vi "Build FIU Section from XML.vi"(6 "Channels":refnum<k24>[](array[refnum]), 8 "error in (no error)":errorcluster, 9 "Card Position in":T1 {"Slot #" max=15}, 10 "Name in":string, 11 "Node Ptr in":u64) -> (0 "error out":errorcluster)   [LabVIEW 2014, in "SLSC configuration System Explorer.lvlib"]
uses:
  SLSC configuration System Explorer.lvlib
  Type Defs/Card Position.ctl
  Shared/SPI Utility/Slot #.ctl
  <vilib>/NI Veristand/Custom Device API/Custom Device Channel.ctl
  <vilib>/NI Veristand/Custom Device API/Custom Device Channel Type.ctl
  Shared/Constants.vi
  <vilib>/NI Veristand/Custom Device API/Set Item Property (U16).vi
  <vilib>/NI Veristand/Custom Device API/Custom Device API.lvlib
  Shared/SLSC configuration Shared.lvlib
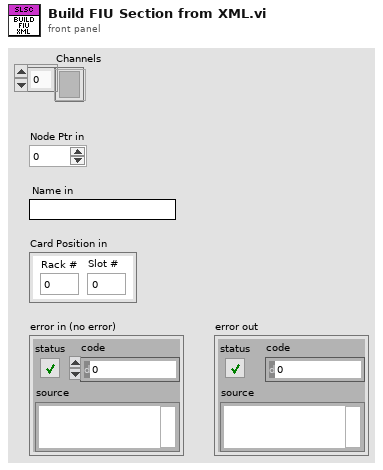
[diagram p1: front panel]
types:
  T1 = typedef "SLSC configuration Shared.lvlib/Card Position.ctl" = cluster{"Rack #":u8, "Slot #":T2}
  T2 = typedef "SLSC configuration Shared.lvlib/Slot #.ctl" = u8
  T3 = typedef "Custom Device API.lvlib/Custom Device Channel Type.ctl" = enum16{"Input", "Output"}
  T4 = typedef "Custom Device API.lvlib/Custom Device Channel.ctl" = cluster{"Type":T3, "Units":string, "Default Value":dbl, "Faultable":bool, "Scalable":bool}
  T5 = typedef "Custom Device API.lvlib/Custom Device Item Ref.ctl" = u64
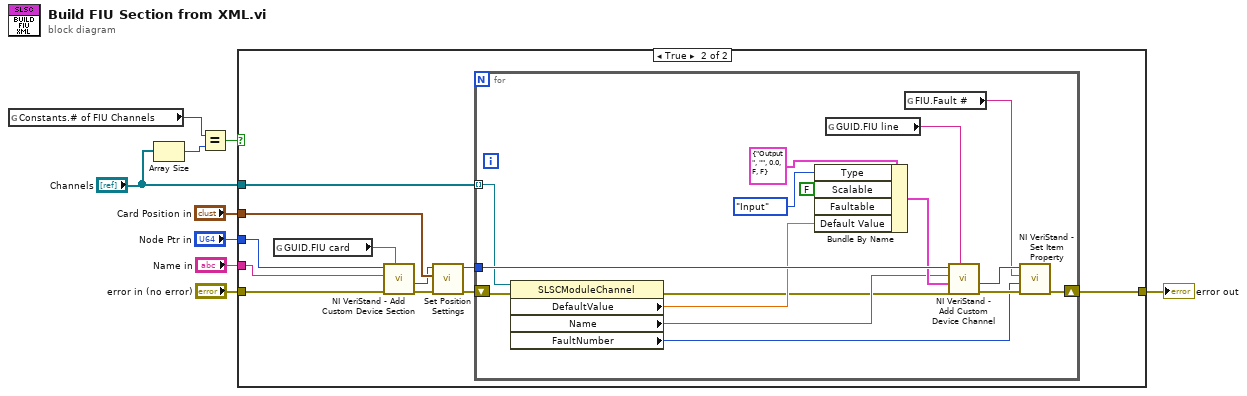
[diagram p0: block diagram]
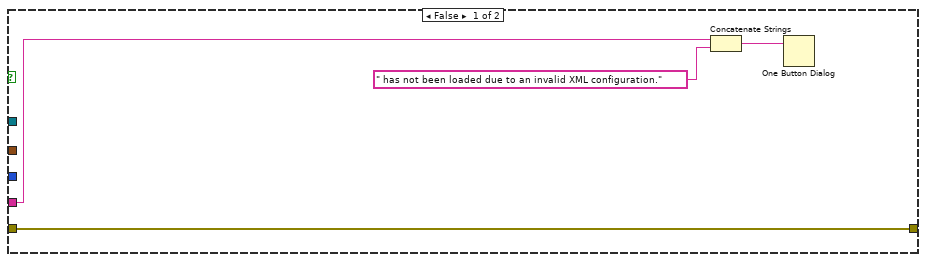
[diagram p2: hidden frame]
diagram:
  n1 = global read "Constants.vi" "Constants.# of FIU Channels"() -> (w2:u8)
  n2 = Array Size(array="Channels") -> (size(s)=w3:i32)
  n3 = Equal?(x=w2, y=w3) -> (x = y?=w4:bool)
  n4 = case shown="True" w4 {
    tunnel: "Node Ptr in" -> [_ w24]
    tunnel: "Name in" -> [w10 w23]
    tunnel: "error in (no error)" -> [w13 w22]
    tunnel: "Card Position in" -> [_ w17]
    tunnel: [w13 w14] -> w9
    tunnel: "Channels" -> [_ w15]
    frame False {
      n5 = Concatenate Strings(w10, " has not been loaded due to an invalid XML configuration." ("string")) -> (w11:string)
      n6 = One Button Dialog(message=w11) -> ()  [unwired: 1 in, 1 out]
    }
    frame True {
      n7 = global read "Constants.vi" "GUID.FIU card"() -> (w21:string)
      n8 = call <vilib>:"NI VeriStand - Add Custom Device Section.vi"("GUID (Default Section)"=w21, "error in (no error)"=w22, "Section Name"=w23, "Parent Ref in"=w24) -> ("error out"=w20:errorcluster, "Section Ptr"=w16:T5)  [unwired: 4 in, 2 out]
      n9 = call "Set Position Settings.vi"("error in (no error)"=w20, "Card Position"=w17, "Item Ref in"=w16) -> ("error out"=w18:errorcluster, "Item Ref out"=w19:T5)  [unwired: 7 in]
      n10 = for {
        shift-right: [w37] -> w14
        shift-left: w18 -> [w29]
        tunnel: w19 -> [w40]
        tunnel: w15 -> [w30] mode=indexing
        w31 = FALSE ("Scalable")
        n11 = property class="SLSCModuleChannel"(reference=w30, error in=w29) -> (error out=w25:errorcluster, "DefaultValue"=w28:dbl, "Name"=w27:string, "FaultNumber"=w26:u8)  [unwired: 1 out]
        n12 = Bundle By Name(cluster=T4 {"Type"=enum."Output", "Units"="", "Default Value"=0.0, "Faultable"=FALSE, "Scalable"=FALSE} ("Channel"), "Type"=Custom_Device_Channel_Type."Input", "Scalable"=w31, "Faultable"=w31, "Default Value"=w28) -> (w33:T4)
        n13 = global read "Constants.vi" "GUID.FIU line"() -> (w39:string)
        n14 = global read "Constants.vi" "FIU.Fault #"() -> (w35:string)
        n15 = call <vilib>:"NI VeriStand - Add Custom Device Channel.vi"("GUID (Default Channel)"=w39, "error in (no error)"=w25, "Channel"=w33, "Channel Name"=w27, "Parent Ref in"=w40) -> ("error out"=w38:errorcluster, "Channel Ref"=w36:T5)  [unwired: 3 in, 2 out]
        n16 = call-poly <vilib>:"NI VeriStand - Set Item Property.vi"("error in (no error)"=w38, "Value"=w26, "Property Name"=w35, "Item Ref in"=w36) -> ("error out"=w37:errorcluster)  [unwired: 5 in, 2 out]
      }
    }
  }
  "error out" <- w9
